vi "ThermoCouple_Logger.vi"() -> ()   [LabVIEW 2024]
uses:
  <vilib>/Platform/TimedLoop/XDataNode/timing_clust.ctl
  <vilib>/Platform/TimedLoop/XDataNode/nitl_modes.ctl
  <vilib>/Platform/TimedLoop/XDataNode/wakeup.ctl
  <extravilib>/ChannelInstances/Tag-c(bool,ref(UserDefinedRefnumTag),bool,path,bool)/Read With Abort.vi
  <extravilib>/ChannelInstances/Tag-c(bool,ref(UserDefinedRefnumTag),bool,path,bool)/Write With Abort.vi
  <extravilib>/ChannelInstances/Tag-c(bool,ref(UserDefinedRefnumTag),bool,path,bool)/Instantiate.vi
  <extravilib>/ChannelInstances/Tag-c(bool,ref(UserDefinedRefnumTag),bool,path,bool)/EndpointRead.vi
  <extravilib>/ChannelInstances/Tag-c(bool,ref(UserDefinedRefnumTag),bool,path,bool)/Endpoint.vi
  <vilib>/platform/TimedLoop/XDataNode/XDataNode.xnode
  <vilib>/Platform/TimedLoop/XDataNode/XDNodeRunTimeDep.lvlib
  <extravilib>/ChannelInstances/Tag-c(bool,ref(UserDefinedRefnumTag),bool,path,bool).lvlib
panel:
  out "Process (ms)":i64
  out "error out 3":errorcluster
  out "error out 2":errorcluster
  in  "samples":i32=10 min=1 max=1000
  in  "Period (ms)":i64=500 min=250 max=2000
  in  "Channel":refnum<k21>
  in  "Start":bool
  out "Temps":waveform(dbl)[](graph)=[{"t0"=timestamp(0 s since 1904-01-01), "dt"=0.5, "Y"=[-0.5459297948238789, -0.5384662523625495, -0.5305055716687722, -0.5227516337304128, -0.5152151485633342, -0.5074594731778411, -0.5000110550794236, -0.49229613528221505, -0.48455544270581347, -0.47704875214651904, -0.4694184221817747, -0.4617297562684411, -0.4542538363910736, -0.44666324774779786, -0.43914993037163397, -0.4315969934450372, -0.42413652957329057, -0.41648702187743, -0.4090503718449979, -0.40158637492342547, -0.3941665018638969, -0.38661414017374235, -0.3792972035366138, -0.37178469009330656, -0.3640722423599955, -0.3568479440776631, -0.3495051306403334, -0.3421642645601655, -0.33493653098477, -0.3275193397439705, -0.32018295336060504, -0.3128894600430486, -0.3055440591103306, -0.29873448073929, -0.29143683883588484, -0.2843423086450982, -0.2772355209388995, -0.27008916517709947, -0.26279625635638254, -0.2557072429162988, -0.24884447893036513, -0.2418962610460262, -0.23471006933283486, -0.22766777081987025, -0.22069024864064335, -0.21390317409486895, -0.20710909597313554, -0.20017922598796378, -0.19328186072145903, -0.18648965958030286, -0.17982101574808698, -0.17308125272085514, -0.16650153019624944, -0.15972005812583243, -0.15288052381799008, -0.14672994680516058, -0.14007374846858675, -0.1336178193214643, -0.12705690492929214, -0.12060549031730709, -0.11444511771368156, -0.10804984536035589, -0.10172786836292154, -0.09532872836465985, -0.08927381125350682, -0.08296971036909855, -0.07689207711853907, -0.07078036829076739, -0.06468688490901309, -0.058868939175738766, -0.05270999822746214, -0.04685361027102993, -0.04104637566433278]}, {"t0"=timestamp(0 s since 1904-01-01), "dt"=0.5, "Y"=[-30.0, -30.0, -30.0, -30.0, -30.0, -30.0, -30.0, -30.0, -30.0, -30.0, -30.0, -30.0, -30.0, -30.0, -30.0, -30.0, -30.0, -30.0, -30.0, -30.0, -30.0, -30.0, -30.0, -30.0, -30.0, -30.0, -30.0, -30.0, -30.0, -30.0, -30.0, -30.0, -30.0, -30.0, -30.0, -30.0, -30.0, -30.0, -30.0, -30.0, -30.0, -30.0, -30.0, -30.0, -30.0, -30.0, -30.0, -30.0, -30.0, -30.0, -30.0, -30.0, -30.0, -30.0, -30.0, -30.0, -30.0, -30.0, -30.0, -30.0, -30.0, -30.0, -30.0, -30.0, -30.0, -30.0, -30.0, -30.0, -30.0, -30.0, -30.0, -30.0, -30.0]}]
  out "Gradients":waveform(dbl)[](graph)
  out "error out":errorcluster
  in  "error in":errorcluster
  out "Status":string="System ready"
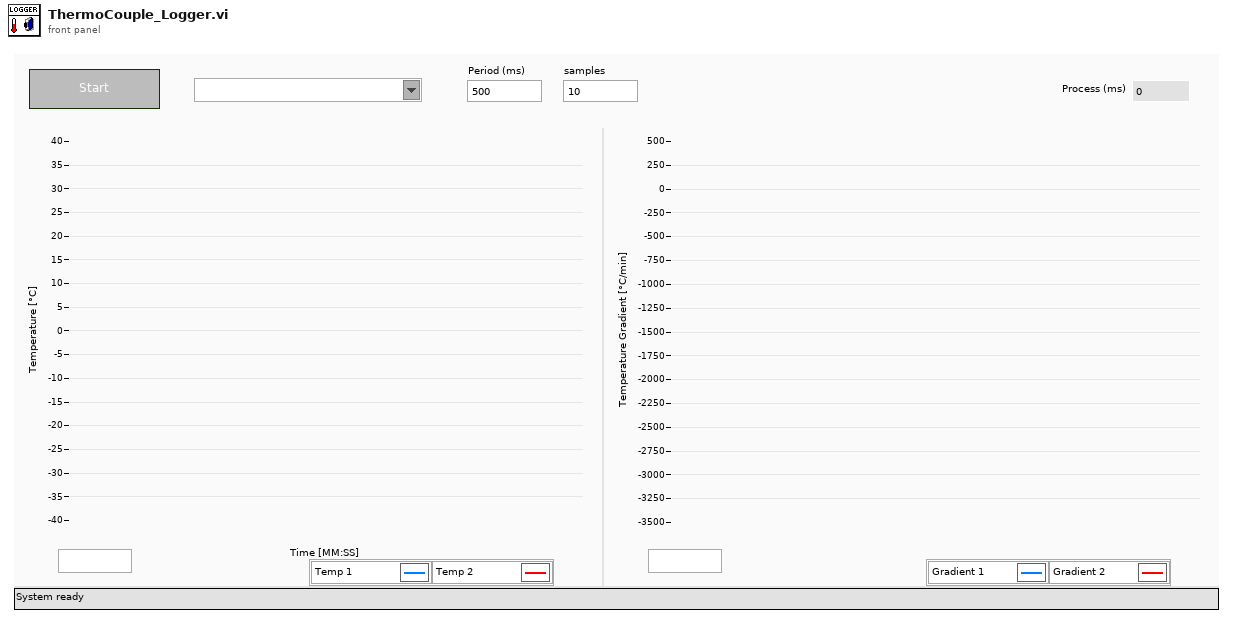
[diagram p1: front panel]
types:
  T1 = cluster{"Active":bool, "task out":refnum<k21>, "Stop":bool, "Path":path, "Connected":bool}
  T2 = enum8{"Enabled", "Disabled", "Disabled and Grayed Out"}
  T3 = typedef "Tag-c(bool,ref(UserDefinedRefnumTag),bool,path,bool).lvlib/))Channel.ctl" = refnum<queue>
  T4 = typedef "XDNodeRunTimeDep.lvlib/timing_clust.ctl" = cluster{"Expected End [f-1]":u64, "Actual End [f-1]":u64, "Finished Late? [f-1]":bool, "Expected End [i-1]":u64, "Actual End [i-1]":u64, "Finished Late? [i-1]":bool, "Expected Start [i]":u64, "Actual Start [i]":u64, "Expected Start [f]":u64, "Actual Start [f]":u64, "Source Name":string, "Structure Name":string, "Period":i64, "Deadline":i64, "Offset":i64, "Start":i64, "Priority":i32, "Timeout":i32, "Mode":T5, "Wakeup Reason":T6, "Error":errorcluster, "Source Type":string, "Secondary Source Type":string, "Global End Time":u64, "Global Start Time":u64, "Frame Duration":u64, "Iteration Duration":u64, "Assigned CPU":i32, "I/O Scan Engine Mode":u32}
  T5 = typedef "XDNodeRunTimeDep.lvlib/nitl_modes.ctl" = enum32{"No Change", "Process missed periods, maintain original phase", "Discard missed periods, maintain original phase", "Process missed periods, ignore original phase", "Discard missed periods, ignore original phase"}
  T6 = typedef "XDNodeRunTimeDep.lvlib/wakeup.ctl" = enum32{"Normal", "Aborted", "Asynchronous wakeup", "Timing source error", "Timed loop error", "Timeout"}
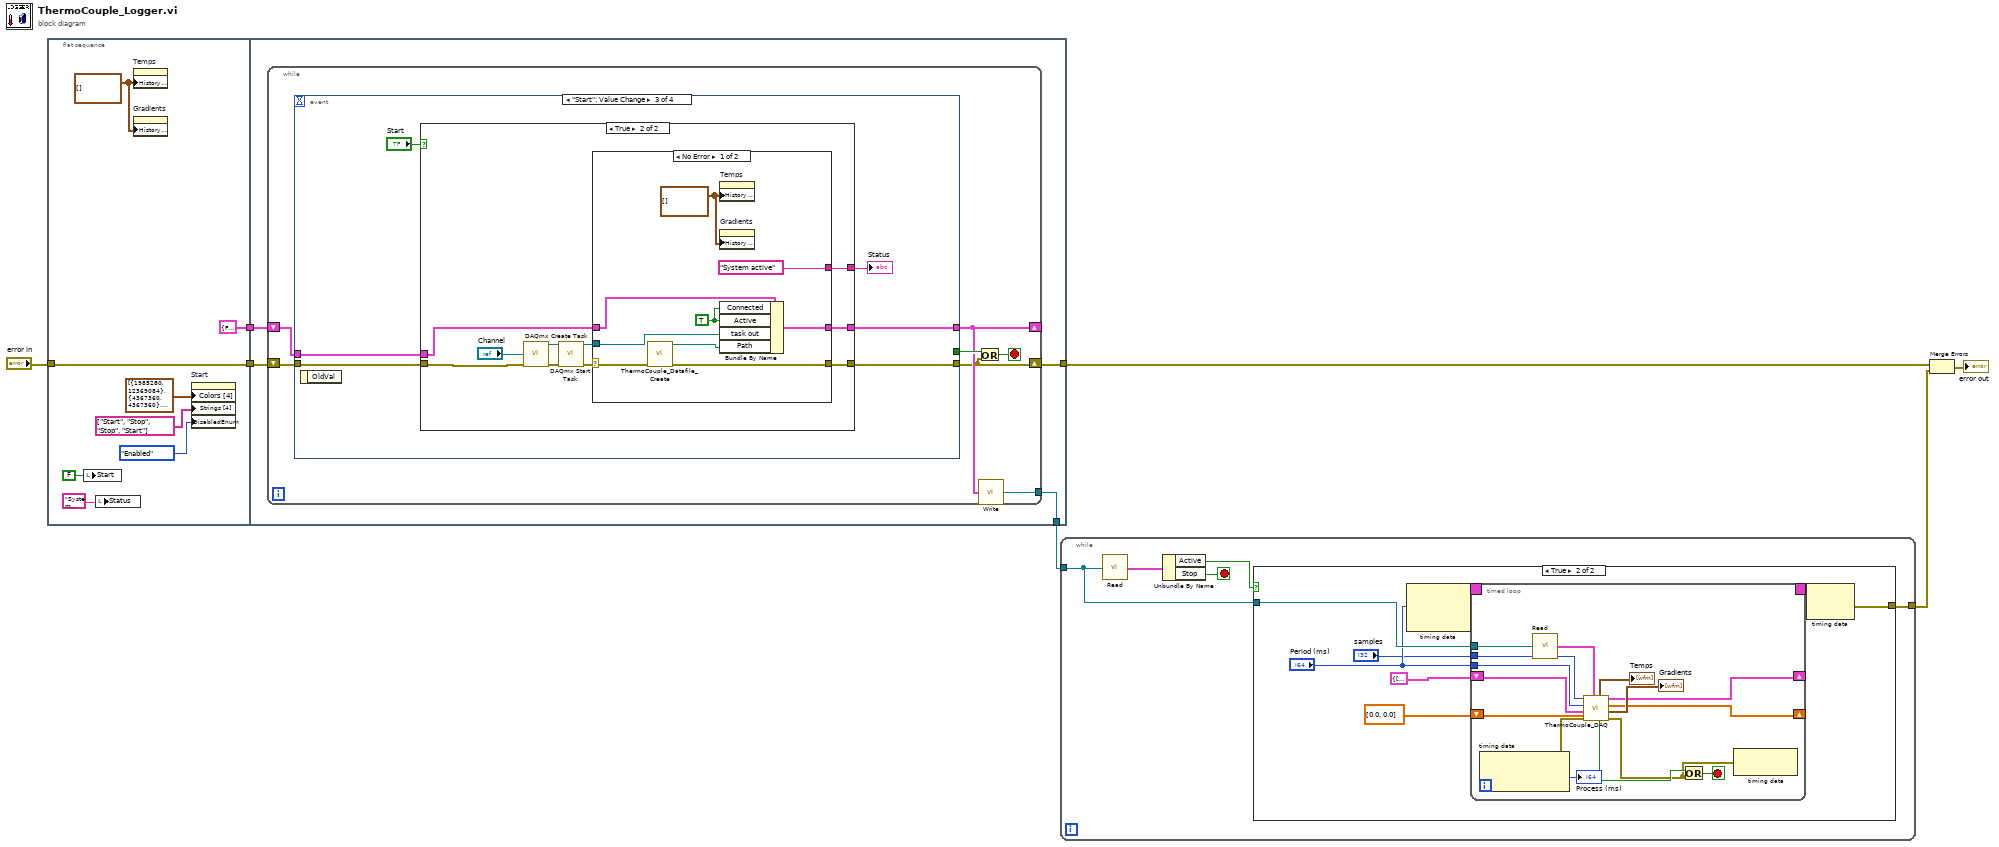
[diagram p0: block diagram]
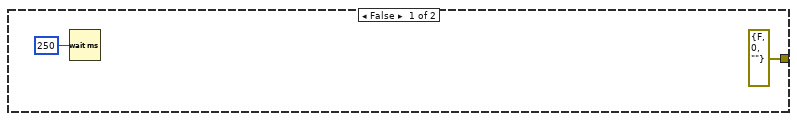
[diagram p2: hidden frame]
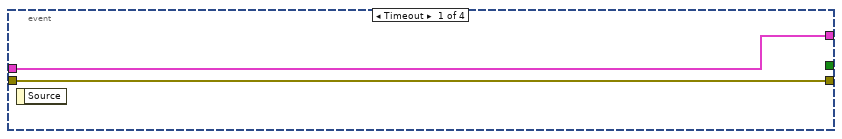
[diagram p3: hidden frame]
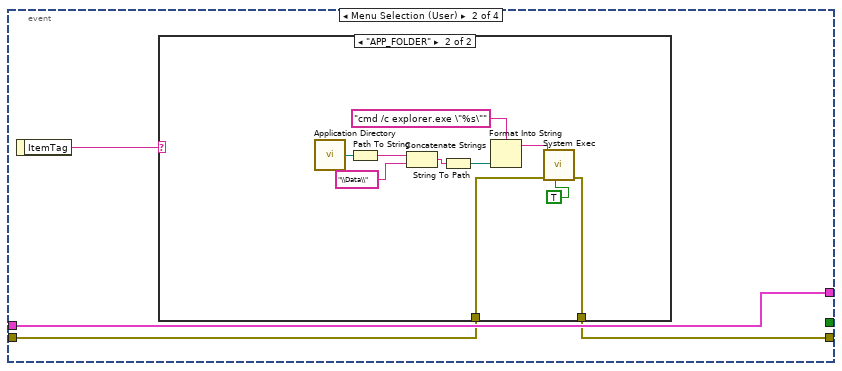
[diagram p4: hidden frame]
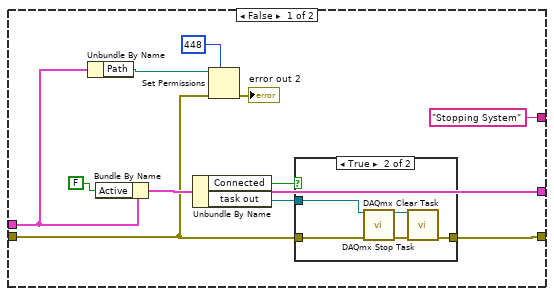
[diagram p6: hidden frame]
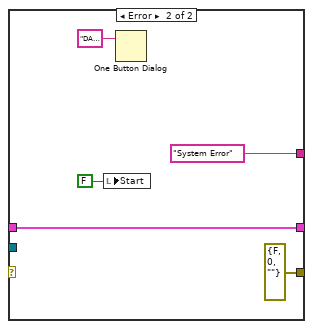
[diagram p8: hidden frame]
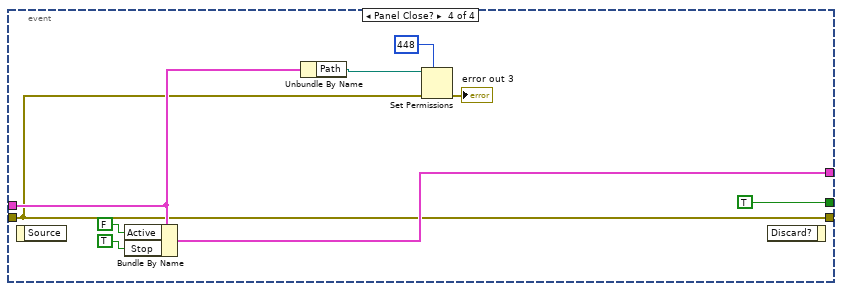
[diagram p9: hidden frame]
diagram:
  n1 = flat-sequence {
    tunnel: [w15] -> w7
    tunnel: "error in" -> [w15]
    tunnel: [T1 {"Active"=FALSE, "task out"="", "Stop"=FALSE, "Path"=path "", "Connected"=FALSE} ("output cluster")] -> w5
    tunnel: w7 -> [w19]
    tunnel: w5 -> [w18]
    tunnel: [w16] -> w1
    tunnel: [w17] -> w4
    frame #0 {
      w13 = waveform(dbl)[][] [] ("History Data")
      n2 = local write "Start"(FALSE ("Accept Values")) -> ()
      n3 = local write "Status"("System Ready" ("Status")) -> ()
      n4 = property on="Temps" class="WFChart (strict)"("History Data"=w13) -> ()  [unwired: 2 in, 2 out]
      n5 = property on="Gradients" class="WFChart (strict)"("History Data"=w13) -> ()  [unwired: 2 in, 2 out]
      n6 = property on="Start" class="Bool (strict)"("Colors [4]"=cluster{u32, u32}[] [{1985280, 12369084}, {4367360, 4367360}, {8388608, 16711681}, {1985280, 1985280}, {1985280, 4367360}, {8388608, 16711681}], "Strings [4]"=string[] ["Start", "Stop", "Stop", "Start"], "DisabledEnum"=T2."Enabled" ("Disabled")) -> ()  [unwired: 2 in, 2 out]
    }
    frame #1 {
      n7 = while {
        shift-right: [w23] -> _
        shift-left: w18 -> [w24]
        tunnel: [w20] -> w16
        shift-right: [w21] -> w17
        shift-left: w19 -> [w22]
        stop <- w25 stop-if-true
        n8 = event shown="[2] \"Start\": Value Change" {
          selector: _ -> [_ _ _ _]
          dyn-events: _ -> [_ _ _ _]
          timeout: _ -> [_ _ _ _]
          tunnel: [_ _ _ TRUE] -> w26
          tunnel: w24 -> [w28 w32 w48 w92]
          tunnel: [w28 w32 w47 w98] -> w23
          tunnel: w22 -> [w27 w30 w46 w91]
          tunnel: [w27 w29 w45 w91] -> w21
          event Timeout {
            n9 = event-data() -> ()  [unwired: 1 in, 1 out]
          }
          event Menu Selection (User) {
            n10 = event-data() -> ("ItemTag"=w31:string)  [unwired: 1 in]
            n11 = case shown="\"APP_FOLDER\"" w31 {
              tunnel: w30 -> [w33 w35]
              tunnel: [w33 w34] -> w29
              frame "False", Default {
              }
              frame "APP_FOLDER" {
                n12 = call <vilib>:"Application Directory.vi"() -> ("Application Directory"=w40:path)
                n13 = Path To String(path=w40) -> (string=w39:string)
                n14 = Concatenate Strings(w39, "\\Data\\") -> (w41:string)
                n15 = String To Path(string=w41) -> (path=w42:path)
                n16 = Format Into String(format string="cmd /c explorer.exe \"%s\"", w42) -> (resulting string=w43:string)  [unwired: 2 in, 1 out]
                n17 = call <vilib>:"System Exec.vi"("run minimized? (F)"=TRUE, "error in (no error)"=w35, "command line"=w43) -> ("error out"=w34:errorcluster)  [unwired: 5 in, 3 out]
              }
            }
          }
          event "Start": Value Change {
            n18 = event-data() -> ()  [unwired: 1 in, 1 out]
            n19 = case shown="True" "Start" {
              tunnel: w48 -> [w57 w75]
              tunnel: [w54 w74] -> w47
              tunnel: ["Stopping System" ("Status") w73] -> w44
              tunnel: w46 -> [w53 w72]
              tunnel: [w52 w71] -> w45
              frame False {
                n20 = Unbundle By Name(w57) -> ("Path"=w56:path)
                n21 = Bundle By Name(cluster=w57, "Active"=FALSE) -> (w54:T1)
                n22 = Unbundle By Name(w54) -> ("Connected"=w50:bool, "task out"=w51:refnum<k21>)
                n23 = Set Permissions(7:i16 448 ("permissions"), 8:w53, 11:w56) -> (0:→"error out 2":errorcluster)  [unwired: 2 in, 1 out]
                n24 = case shown="True" w50 {
                  tunnel: w51 -> [_ w66]
                  tunnel: w53 -> [w61 w65]
                  tunnel: [w61 w62] -> w52
                  frame False {
                  }
                  frame True {
                    n25 = call <vilib>:"DAQmx Stop Task.vi"("task/channels in"=w66, "error in"=w65) -> ("task out"=w63:refnum<k21>, "error out"=w64:errorcluster)  [unwired: 12 in]
                    n26 = call <vilib>:"DAQmx Clear Task.vi"("task in"=w63, "error in"=w64) -> ("error out"=w62:errorcluster)  [unwired: 13 in]
                  }
                }
              }
              frame True {
                n27 = call <vilib>:"DAQmx Create Task.vi"("global virtual channels"="Channel", "error in"=w72) -> ("task out"=w70:refnum<k21>, "error out"=w69:errorcluster)  [unwired: 12 in]
                n28 = call <vilib>:"DAQmx Start Task.vi"("task/channels in"=w70, "error in"=w69) -> ("task out"=w67:refnum<k21>, "error out"=w68:errorcluster)  [unwired: 12 in]
                n29 = case shown="No Error" w68 {
                  selector: w68 -> [w82 _]
                  tunnel: w67 -> [w79 _]
                  tunnel: w75 -> [w85 w89]
                  tunnel: [w84 w89] -> w74
                  tunnel: ["System active" ("Status") "System Error" ("Status")] -> w73
                  tunnel: [w81 errorcluster {"status"=FALSE, "code"=0, "source"=""} ("error out")] -> w71
                  frame No Error {
                    w78 = waveform(dbl)[][] [] ("History Data")
                    w77 = TRUE ("Active")
                    n30 = call "ThermoCouple_Datafile_Create.vi"("error in (no error)"=w82) -> ("error out"=w81:errorcluster, "path out"=w80:path)  [unwired: 9 in]
                    n31 = property on="Temps" class="WFChart (strict)"("History Data"=w78) -> ()  [unwired: 2 in, 2 out]
                    n32 = property on="Gradients" class="WFChart (strict)"("History Data"=w78) -> ()  [unwired: 2 in, 2 out]
                    n33 = Bundle By Name(cluster=w85, "Connected"=w77, "Active"=w77, "task out"=w79, "Path"=w80) -> (w84:T1)
                  }
                  frame Error {
                    n34 = local write "Start"(FALSE ("Start")) -> ()
                    n35 = One Button Dialog(message="DAQ Channel Failed") -> ()  [unwired: 1 in, 1 out]
                  }
                }
              }
            }
            "Status" <- w44
          }
          event Panel Close? {
            n36 = event-data() -> ()  [unwired: 1 in, 1 out]
            n37 = Bundle By Name(cluster=w92, "Active"=FALSE, "Stop"=TRUE) -> (w98:T1)
            n38 = Unbundle By Name(w92) -> ("Path"=w94:path)
            n39 = Set Permissions(7:i16 448 ("permissions"), 8:w91, 11:w94) -> (0:→"error out 3":errorcluster)  [unwired: 2 in, 1 out]
            n40 = event-data() -> ()  [unwired: 2 in, 1 out]
          }
        }
        n41 = Or(x=w26, y=w21) -> (x .or. y?=w25:bool)
        n42 = call <extravilib>:"Write.vi"("element"=w23) -> ("channel"=w20:T3)  [unwired: 1 out]
      }
    }
  }
  n43 = while {
    tunnel: [w104] -> w3
    tunnel: w1 -> [w100]
    stop <- w101 stop-if-true
    n44 = call <extravilib>:"Read.vi"("channel"=w100) -> ("element"=w102:T1)  [unwired: 1 in, 1 out]
    n45 = Unbundle By Name(w102) -> ("Active"=w103:bool, "Stop"=w101:bool)
    n46 = case shown="True" w103 {
      tunnel: [errorcluster {"status"=FALSE, "code"=0, "source"=""} ("Error") w112] -> w104
      tunnel: w100 -> [_ w111]
      frame False {
        n47 = Wait (ms)(milliseconds to wait=u32 250) -> ()  [unwired: 1 out]
      }
      frame True {
        n48 = node-c288("Period (ms)") -> (w114:T4)  [unwired: 1 in]
        n49 = timed-loop {
          timing: w114 -> [_]
          timing-out: [_] -> w113
          shift-right: [w123] -> _
          shift-left: cluster{"Temps":dbl[][], "Gradients":dbl[][]} {"Temps"=[[0.0], [0.0]], "Gradients"=[[0.0], [0.0]]} ("Data out") -> [w122]
          tunnel: w111 -> [w128]
          tunnel: "Period (ms)" -> [w121]
          tunnel: "samples" -> [w120]
          shift-right: [w116] -> _
          shift-left: dbl[] [0.0, 0.0] ("Temps out") -> [w119]
          stop <- w129 stop-if-true
          n50 = node-c288() -> (w118:errorcluster, →"Process (ms)":i64)  [unwired: 1 in]
          n51 = call <extravilib>:"Read.vi"("channel"=w128) -> ("element"=w127:T1)  [unwired: 1 in, 1 out]
          n52 = call "ThermoCouple_DAQ.vi"("Temps in"=w119, "Setup"=w127, "error in (no error)"=w118, "Data in"=w122, "Period (ms)"=w121, "samples"=w120) -> ("error out"=w117:errorcluster, "Gradients graph"=→"Gradients":waveform(dbl)[], "Temps out"=w116:dbl[], "Data out"=w123:cluster{"Temps":dbl[][], "Gradients":dbl[][]}, "stop?"=w126:bool, "Temps graph"=→"Temps":waveform(dbl)[])
          n53 = Or(x=w126, y=w117) -> (x .or. y?=w129:bool)
          n54 = node-c288(w117) -> ()  [unwired: 1 out]
        }
        n55 = node-c288(w113) -> (w112:errorcluster)
      }
    }
  }
  n56 = Merge Errors(w4, w3) -> (→"error out":errorcluster)
